vi "test variant to json bool.vi"(8 "error in (no error)":errorcluster) -> (0 "error out":errorcluster)   [LabVIEW 2019, in "labview_json_tests.lvlib"]
uses:
  labview_json_tests.lvlib
  lib/labview_json.lvlib
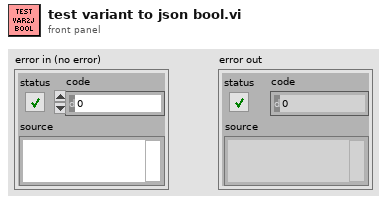
[diagram p1: front panel]
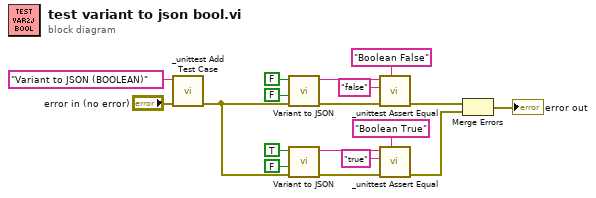
[diagram p0: block diagram]
diagram:
  n1 = call "_unittest Add Test Case.vi"("error in (no error)"="error in (no error)", "Test Case"="Variant to JSON (BOOLEAN)") -> ("error out"=w3:errorcluster)  [unwired: 9 in]
  n2 = call "Variant to JSON.vi"("error in (no error)"=w3, "Pretty Print? (F)"=FALSE, "Variant in"=FALSE) -> ("error out"=w11:errorcluster, "JSON"=w9:string)  [unwired: 7 in]
  n3 = call "Variant to JSON.vi"("error in (no error)"=w3, "Pretty Print? (F)"=FALSE, "Variant in"=TRUE) -> ("error out"=w7:errorcluster, "JSON"=w6:string)  [unwired: 7 in]
  n4 = call "_unittest Assert Equal.vi"("Message"="Boolean False", "error in (no error)"=w11, "Expected Value"="false", "Actual Value"=w9) -> ("error out"=w16:errorcluster)  [unwired: 7 in]
  n5 = call "_unittest Assert Equal.vi"("Message"="Boolean True", "error in (no error)"=w7, "Expected Value"="true", "Actual Value"=w6) -> ("error out"=w12:errorcluster)  [unwired: 7 in]
  n6 = Merge Errors(w16, w12) -> (→"error out":errorcluster)
